vi "Display Biometry Average.vi"(8 "错误常量 2":errorcluster caption="错误常量", 10 "Measure_No":i32, 11 "connection reference":T1) -> (0 "错误常量":errorcluster)   [LabVIEW 2015, in "Browse.lvlib"]
uses:
  Browse.lvlib
  <vilib>/addons/database/Connection.llb/Conn ObjectReference.ctl
  Support/Biometry Average UI Data.ctl
  Support/Display Biometry Average State.ctl
  Sub VIs/Database Processing/Database Processing.lvlib
  <vilib>/addons/database/NI_Database_API.lvlib
  Sub VIs/Utility VIs/Utility VIs.lvlib
panel:
  out "OD":string[][](table)
  out "OS":string[][](table)
  in  "停止按钮":bool
  out "状态栏":string
  # "患者眼球参数浏览"
  # "OD（右眼）"
  # "OS（左眼）"
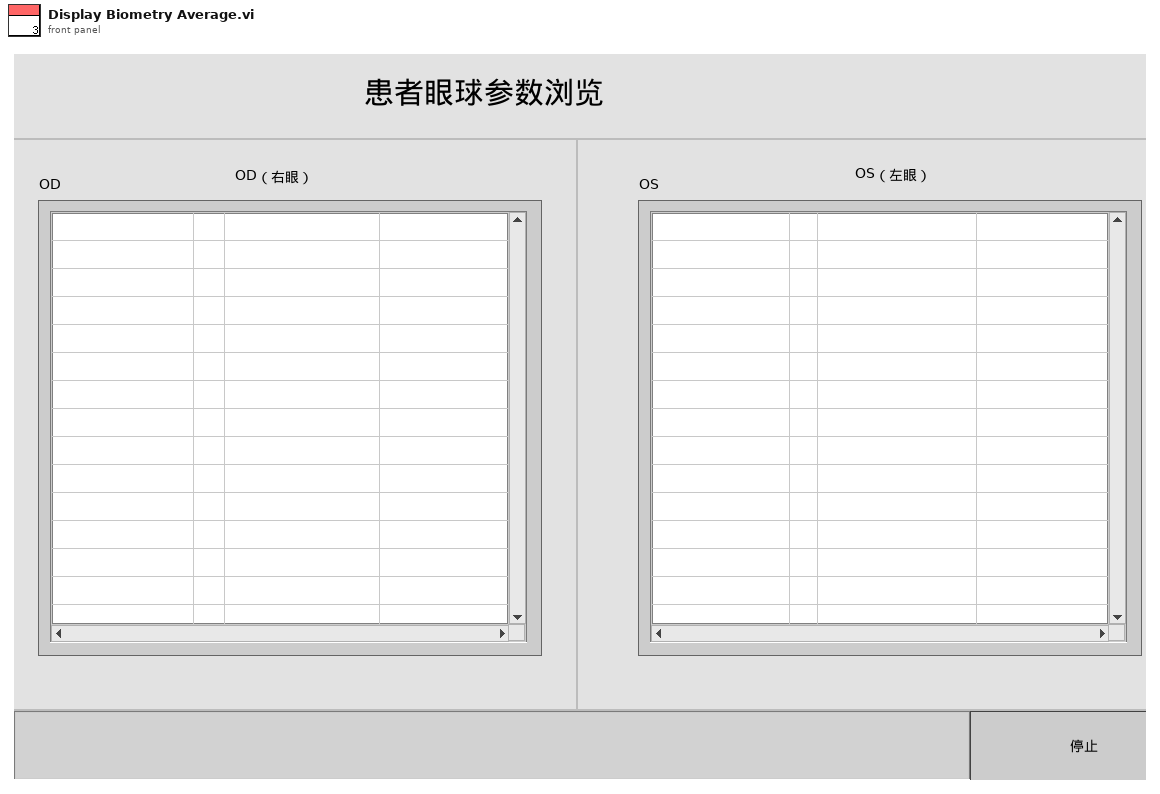
[diagram p1: front panel]
types:
  T1 = typedef "NI_Database_API.lvlib/Conn ObjectReference.ctl" = refnum<k1>
  T2 = typedef "Browse.lvlib/Display Biometry Average State.ctl" = enum16{"Initialize", "Connect Database", "Display Biometry Ascan", "Display Biometry PD Image", "Display Biometry WTW Image", "Display Biometry Keratometric Image", "Update Biometry Average", "Wait For Event", "Exit"}
  T3 = typedef "Browse.lvlib/Biometry Average UI Data.ctl" = cluster{"OD引用句柄":refnum<vi>, "OS引用句柄":refnum<vi>, "状态栏引用句柄":refnum<vi>, "退出引用句柄":refnum<vi>}
  T4 = typedef "LVPoint32TypeDef.ctl" = cluster{"Horizontal":i32, "Vertical":i32}
  T5 = typedef "LVRowAndColumnTypeDef.ctl" = cluster{"Row":i32, "Column":i32}
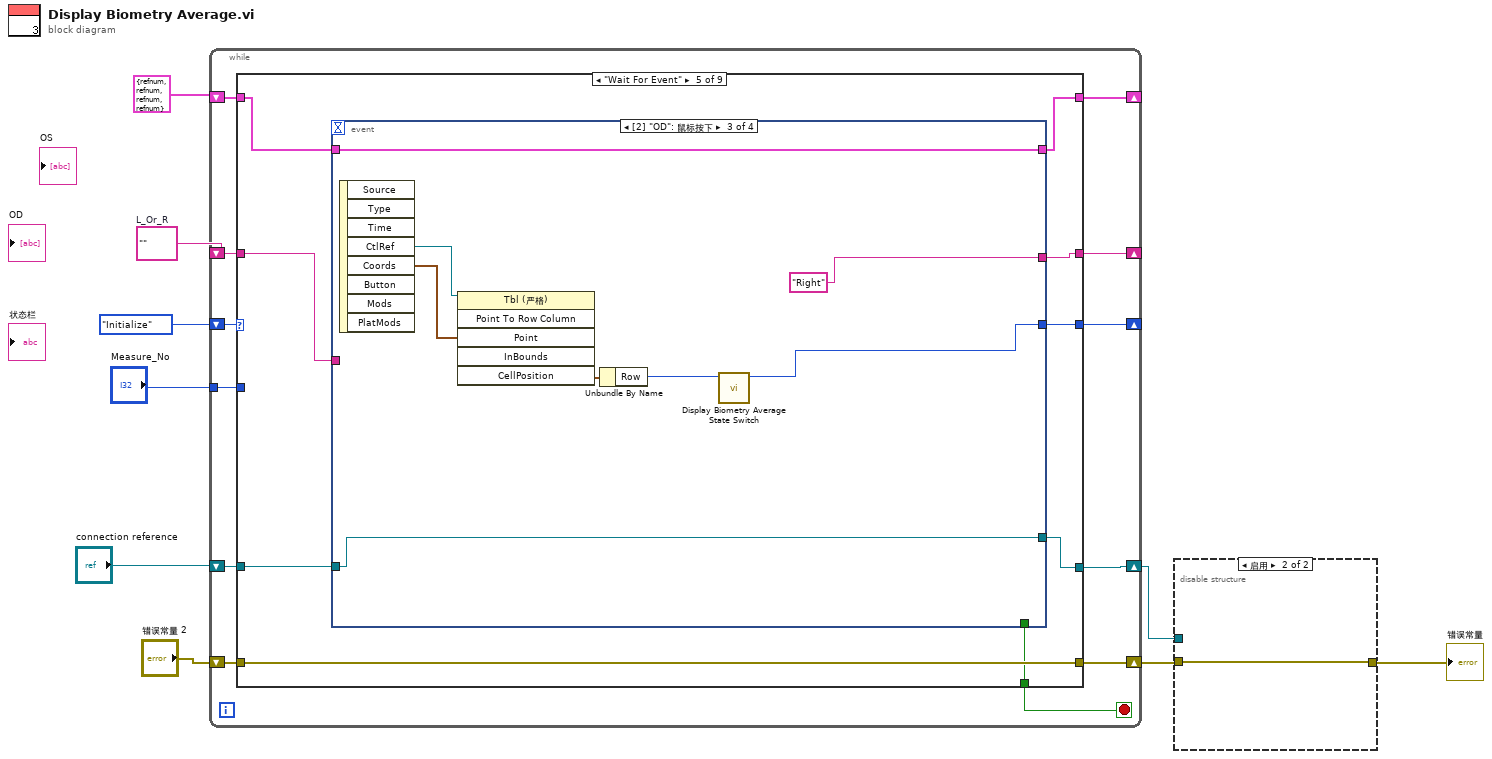
[diagram p0: block diagram]
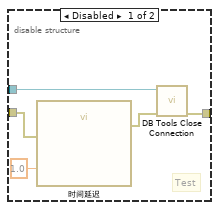
[diagram p2: hidden frame]
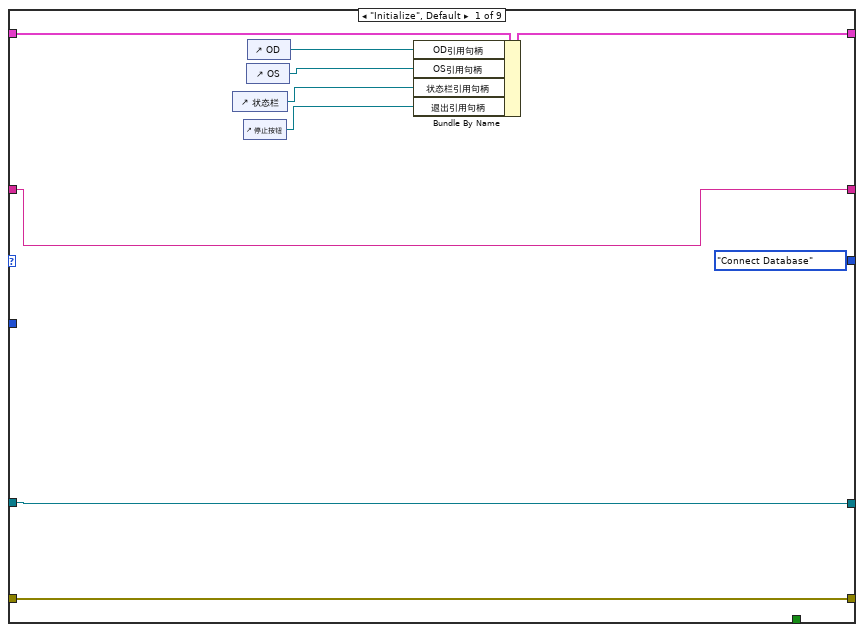
[diagram p3: hidden frame]
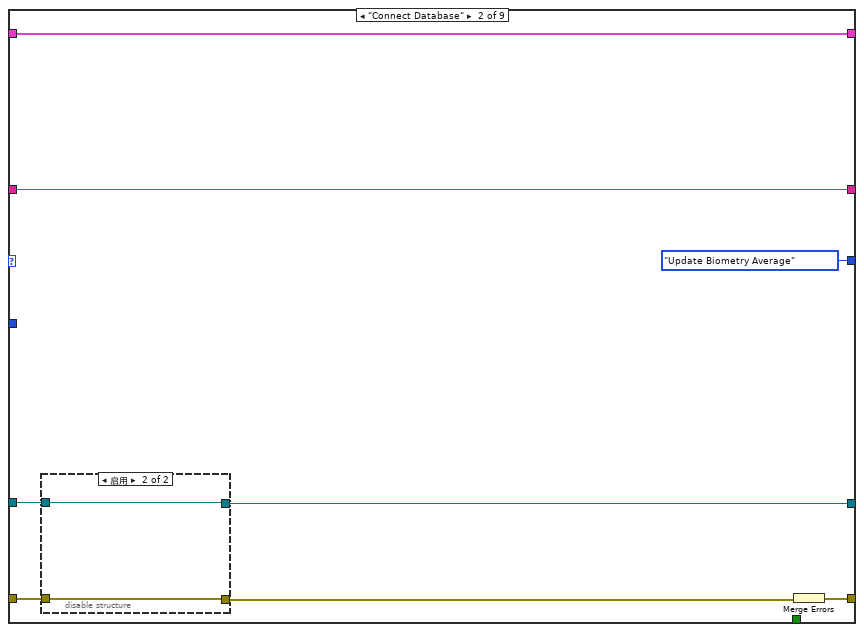
[diagram p4: hidden frame]
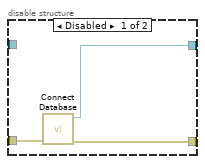
[diagram p5: hidden frame]
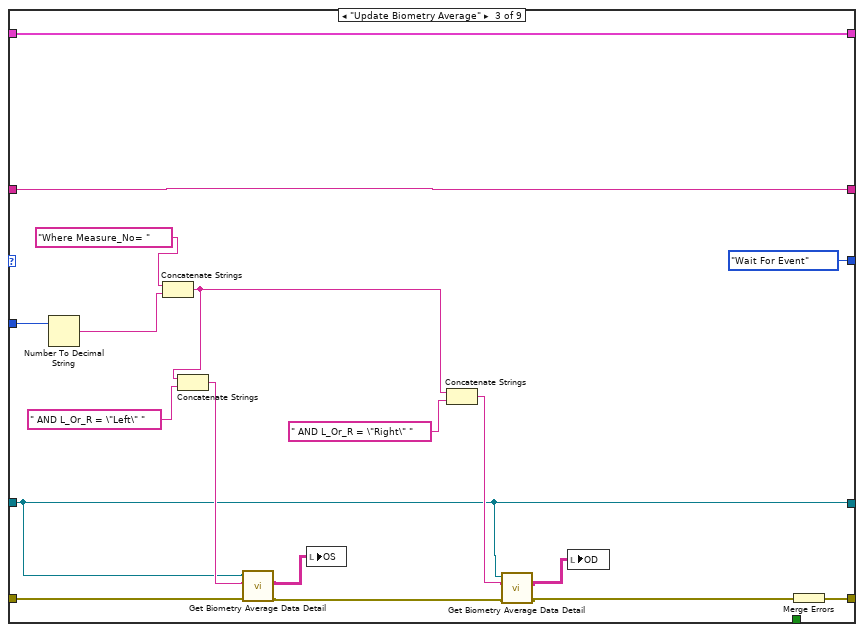
[diagram p6: hidden frame]
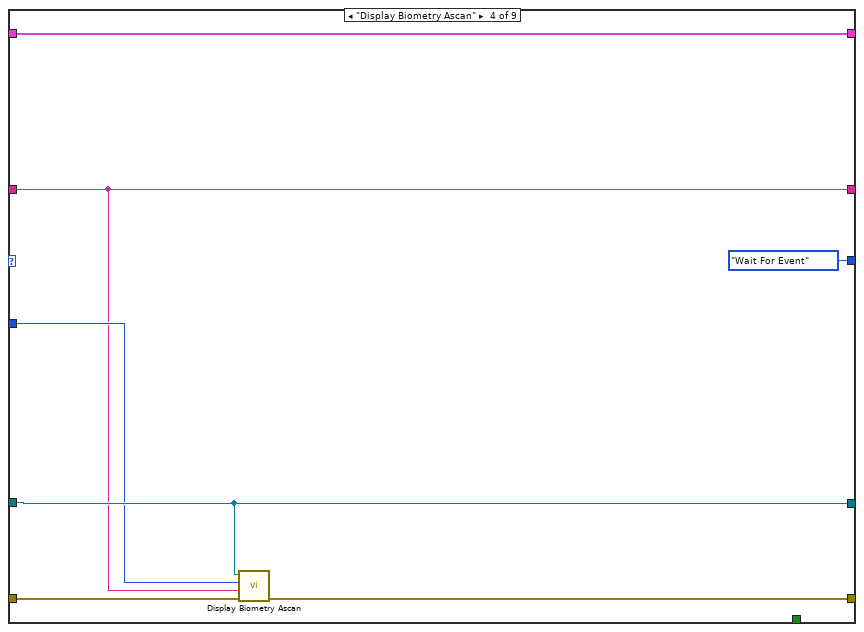
[diagram p7: hidden frame]
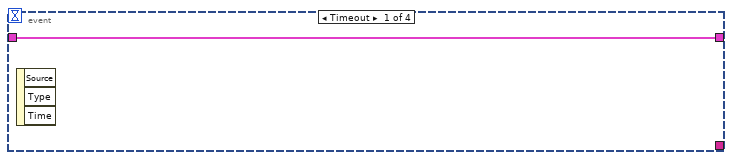
[diagram p8: hidden frame]
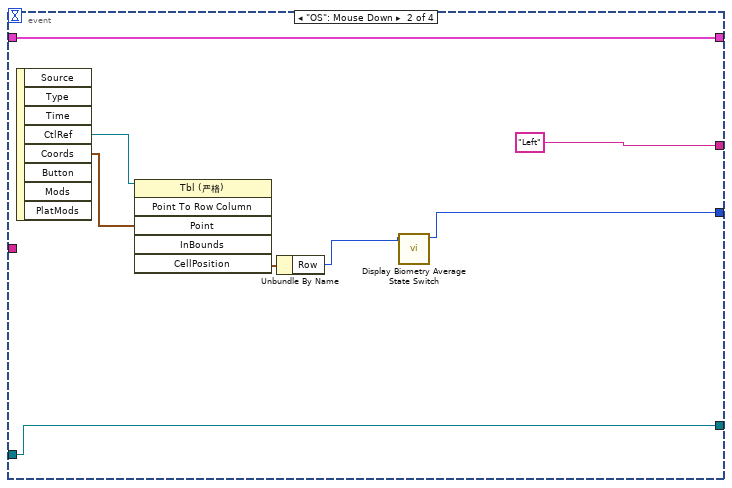
[diagram p9: hidden frame]
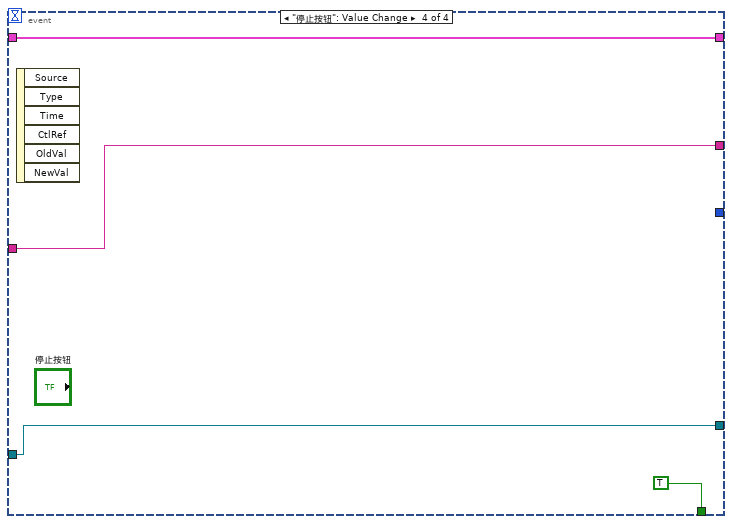
[diagram p10: hidden frame]
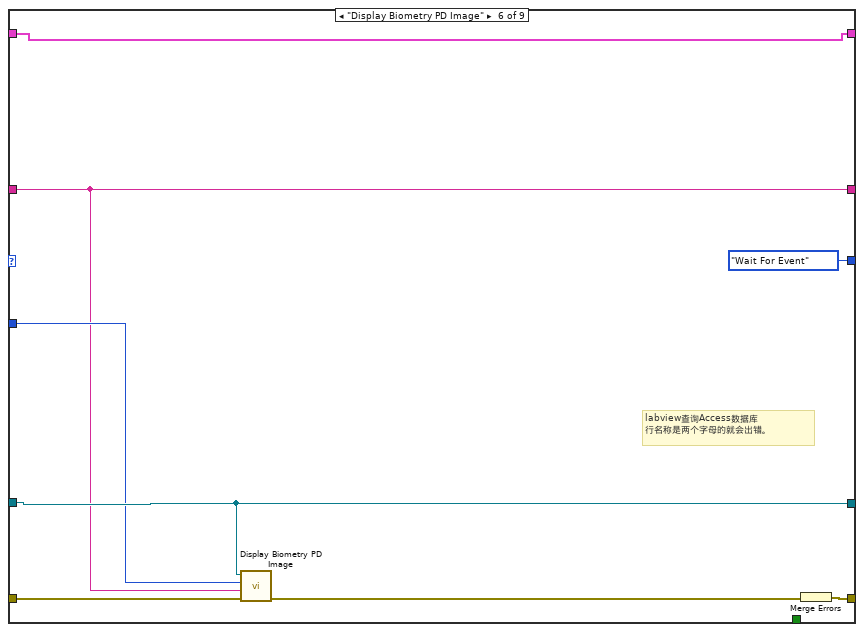
[diagram p11: hidden frame]
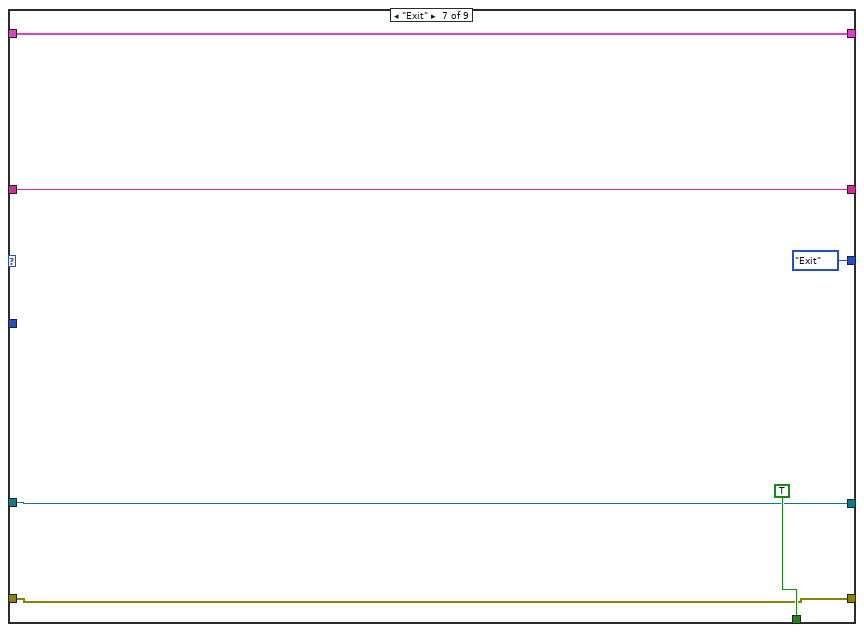
[diagram p12: hidden frame]
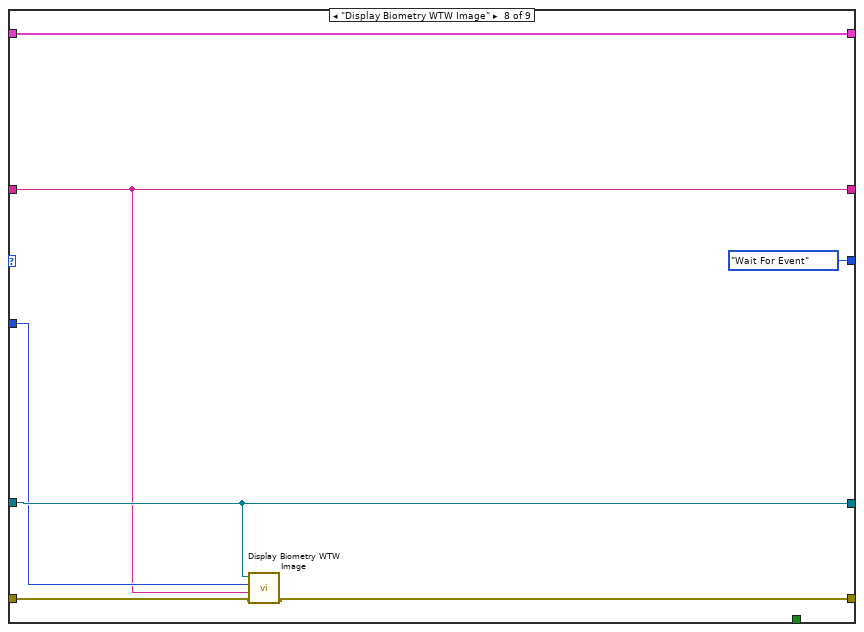
[diagram p13: hidden frame]
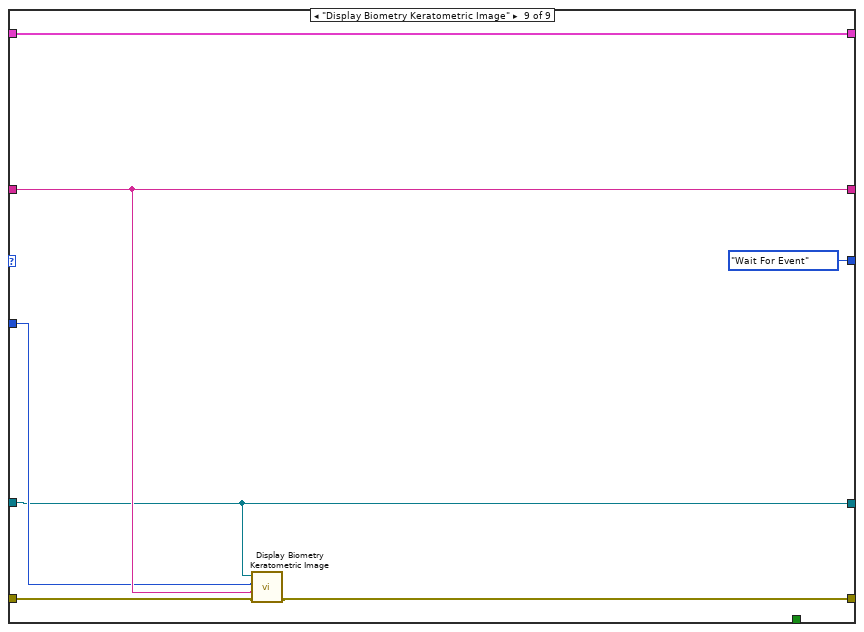
[diagram p14: hidden frame]
diagram:
  w7 = ""  # L_Or_R
  n1 = while {
    shift-right: [w20] -> _
    shift-left: T3 {"OD引用句柄"=refnum, "OS引用句柄"=refnum, "状态栏引用句柄"=refnum, "退出引用句柄"=refnum} ("UI数据") -> [w21]
    shift-right: [w12] -> _
    shift-left: Display_Biometry_Average_State."Initialize" ("State") -> [w11]
    shift-right: [w17] -> w5
    shift-left: "错误常量 2" -> [w19]
    shift-right: [w15] -> _
    shift-left: w7 -> [w18]
    shift-right: [w14] -> w4
    shift-left: "connection reference" -> [w13]
    tunnel: "Measure_No" -> [w10]
    stop <- w16 stop-if-true
    n2 = case shown="\"Wait For Event\"" w11 {
      tunnel: w21 -> [w31 w34 w61 w69 w74 w106 w113 w120 w127]
      tunnel: [w30 w34 w61 w69 w73 w106 w113 w120 w127] -> w20
      tunnel: [Display_Biometry_Average_State."Connect Database" ("State") Display_Biometry_Average_State."Update Biometry Average" ("State") Display_Biometry_Average_State."Wait For Event" ("State") Display_Biometry_Average_State."Wait For Event" ("State") w76 Display_Biometry_Average_State."Wait For Event" ("State") Display_Biometry_Average_State."Exit" ("State") Display_Biometry_Average_State."Wait For Event" ("State") Display_Biometry_Average_State."Wait For Event" ("State")] -> w12
      tunnel: w19 -> [w29 w38 w53 w68 w75 w105 w110 w119 w125]
      tunnel: w18 -> [w28 w35 w59 w64 w78 w101 w112 w115 w123]
      tunnel: [w29 w39 w62 w67 w75 w107 w110 w118 w124] -> w17
      tunnel: [w28 w35 w59 w64 w77 w101 w112 w115 w123] -> w15
      tunnel: [_ _ _ _ w70 _ TRUE _ _] -> w16
      tunnel: w13 -> [w27 w33 w48 w66 w72 w103 w109 w117 w121]
      tunnel: [w27 w36 w48 w66 w71 w103 w109 w117 w121] -> w14
      tunnel: w10 -> [_ _ w57 w65 _ w102 _ w116 w122]
      frame "Initialize", Default {
        n3 = control-ref of="状态栏"() -> (w24:refnum<vi>)
        n4 = control-ref of="停止按钮"() -> (w23:refnum<vi>)
        n5 = control-ref of="OS"() -> (w25:refnum<vi>)
        n6 = control-ref of="OD"() -> (w26:refnum<vi>)
        n7 = Bundle By Name(cluster=w31, "OD引用句柄"=w26, "OS引用句柄"=w25, "状态栏引用句柄"=w24, "退出引用句柄"=w23) -> (w30:T3)
      }
      frame "Connect Database" {
        n8 = disable-structure shown="启用" {
          disable-tunnel: w38 -> [w42 w43]
          disable-tunnel: [w41 w43] -> w37
          disable-tunnel: [w40 w44] -> w36
          disable-tunnel: w33 -> [_ w44]
          frame Disabled {
            n9 = call "Connect Database.vi"("error in (no error)"=w42) -> ("error out"=w41:errorcluster, "connection reference"=w40:T1)  [unwired: 9 in]
          }
          frame Enabled {
          }
        }
        n10 = Merge Errors(w37) -> (w39:errorcluster)
      }
      frame "Update Biometry Average" {
        n11 = Number To Decimal String(number=w57) -> (decimal integer string=w55:string)  [unwired: 1 in]
        n12 = Concatenate Strings("Where Measure_No= " ("字符串"), w55) -> (w54:string)
        n13 = Concatenate Strings(w54, " AND L_Or_R = \"Left\" " ("字符串")) -> (w52:string)
        n14 = call "Get Biometry Average Data Detail.vi"("error in (no error)"=w53, "condition"=w52, "connection reference"=w48) -> ("error out"=w50:errorcluster, "Data Output"=w51:string[][])  [unwired: 7 in]
        n15 = local write "OS"(w51) -> ()
        n16 = Concatenate Strings(w54, " AND L_Or_R = \"Right\" " ("字符串")) -> (w49:string)
        n17 = call "Get Biometry Average Data Detail.vi"("error in (no error)"=w50, "condition"=w49, "connection reference"=w48) -> ("error out"=w46:errorcluster, "Data Output"=w47:string[][])  [unwired: 7 in]
        n18 = local write "OD"(w47) -> ()
        n19 = Merge Errors(w46) -> (w62:errorcluster)
      }
      frame "Display Biometry Ascan" {
        n20 = call "Display Biometry Ascan.vi"("错误常量"=w68, "L_Or_R"=w64, "Measure_No"=w65, "connection reference"=w66) -> ("error out"=w67:errorcluster)  [unwired: 7 in]
      }
      frame "Wait For Event" {
        n21 = event shown="[2] \"OD\": 鼠标按下" {
          selector: _ -> [_ _ _ _]
          dyn-events: _ -> [_ _ _ _]
          timeout: _ -> [_ _ _ _]
          tunnel: w78 -> [_ _ _ w99]
          tunnel: [_ "Left" ("字符串") "Right" ("L_Or_R") w99] -> w77
          tunnel: [_ w80 w88 _] -> w76
          tunnel: w74 -> [w79 w86 w94 w98]
          tunnel: [w79 w86 w94 w98] -> w73
          tunnel: w72 -> [_ w85 w93 w97]
          tunnel: [_ w85 w93 w97] -> w71
          tunnel: [_ _ _ TRUE] -> w70
          event Timeout {
            n22 = event-data() -> ()  [unwired: 1 in, 3 out]
          }
          event "OS": Mouse Down {
            n23 = event-data() -> ("CtlRef"=w83:refnum<vi>, "Coords"=w82:T4)  [unwired: 1 in, 6 out]
            n24 = invoke on="调用节点" class="Tbl (严格)" method="Point To Row Column"(reference=w83, "Point"=w82) -> ("CellPosition"=w87:T5)  [unwired: 4 in, 5 out]
            n25 = Unbundle By Name(w87) -> ("Row"=w81:i32)
            n26 = call "Display Biometry Average State Switch.vi"("Switch"=w81) -> ("State"=w80:T2)  [unwired: 10 in]
          }
          event "OD": Mouse Down {
            n27 = event-data() -> ("CtlRef"=w92:refnum<vi>, "Coords"=w91:T4)  [unwired: 1 in, 6 out]
            n28 = invoke on="调用节点" class="Tbl (严格)" method="Point To Row Column"(reference=w92, "Point"=w91) -> ("CellPosition"=w95:T5)  [unwired: 4 in, 5 out]
            n29 = Unbundle By Name(w95) -> ("Row"=w89:i32)
            n30 = call "Display Biometry Average State Switch.vi"("Switch"=w89) -> ("State"=w88:T2)  [unwired: 10 in]
          }
          event "停止按钮": Value Change {
            n31 = event-data() -> ()  [unwired: 1 in, 6 out]
          }
        }
      }
      frame "Display Biometry PD Image" {
        # "labview查询Access数据库\n行名称是两个字母的就会出错。"
        n32 = call "Display Biometry PD Image.vi"("错误常量"=w105, "L_Or_R"=w101, "Measure_No"=w102, "connection reference"=w103) -> ("error out"=w104:errorcluster)  [unwired: 7 in]
        n33 = Merge Errors(w104) -> (w107:errorcluster)
      }
      frame "Exit" {
      }
      frame "Display Biometry WTW Image" {
        n34 = call "Display Biometry WTW Image.vi"("错误常量"=w119, "L_Or_R"=w115, "Measure_No"=w116, "connection reference"=w117) -> ("error out"=w118:errorcluster)  [unwired: 7 in]
      }
      frame "Display Biometry Keratometric Image" {
        n35 = call "Display Biometry Keratometric Image.vi"("错误常量"=w125, "L_Or_R"=w123, "Measure_No"=w122, "connection reference"=w121) -> ("error out"=w124:errorcluster)  [unwired: 7 in]
      }
    }
  }
  n36 = disable-structure shown="启用" {
    disable-tunnel: w5 -> [w130 w133]
    disable-tunnel: [w132 w133] -> w3
    disable-tunnel: w4 -> [w131 _]
    frame Disabled {
      # "Test"
      n37 = call "时间延迟"("error in (no error)"=w130, "Delay Time (s)"=1.0) -> ("error out"=w129:errorcluster)  [unwired: 9 in]
      n38 = call <vilib>:"DB Tools Close Connection.vi"("error in (no error)"=w129, "connection reference"=w131) -> ("error out"=w132:errorcluster)  [unwired: 5 in]
    }
    frame Enabled {
    }
  }
  "错误常量" <- w3
